vi "Get Channel Name.vi"(8 "error in (no error)":errorcluster, 10 "index":i32, 11 "Impulse Data in":T1) -> (0 "error out":errorcluster, 2 "Channel Name":string, 3 "Impulse Data out":T1)   [LabVIEW 2016, in "Impulse Data.lvclass"]
uses:
  Impulse Data.lvclass
  Instance handle.ctl
  Impulse Data.lvclass/Impulse Data.ctl
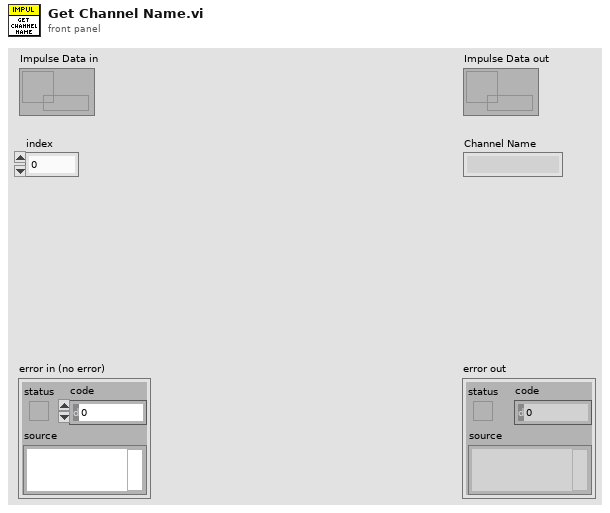
[diagram p1: front panel]
types:
  T1 = typedef "Impulse Data.lvclass/Instance handle.ctl" = refnum<data-value>
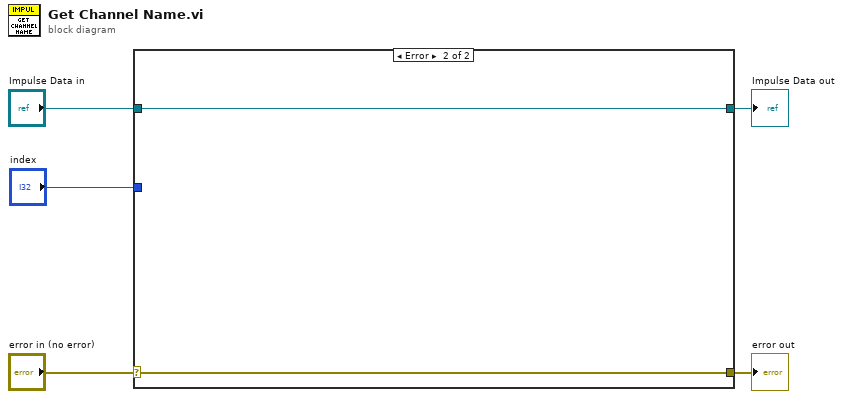
[diagram p0: block diagram]
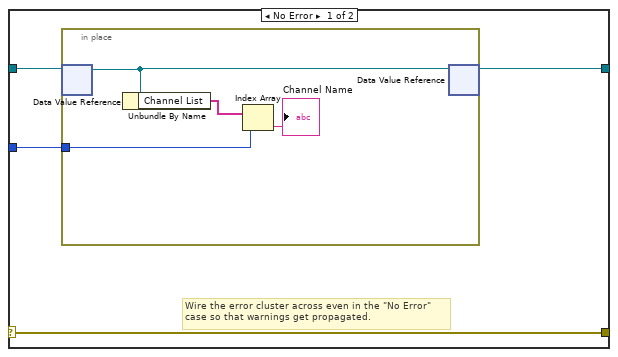
[diagram p2: hidden frame]
diagram:
  n1 = case shown="Error" "error in (no error)" {
    selector: "error in (no error)" -> [w9 w15]
    tunnel: [w9 w15] -> w4
    tunnel: "index" -> [w8 _]
    tunnel: [w7 w14] -> w2
    tunnel: "Impulse Data in" -> [w6 w14]
    frame No Error {
      # "Wire the error cluster across even in the \"No Error\"\ncase so that warnings get propagated."
      n2 = in-place {
        in-place-border: w8 -> [w12]
        n3 = in-place-dvr #1(w6) -> (w10:refnum<class "Impulse Data.lvclass">)  [unwired: 1 out]
        n4 = Unbundle By Name(w10) -> ("Channel List"=w13:string[])
        n5 = Index Array(array=w13, index=w12) -> (element=→"Channel Name":string)
        n6 = in-place-dvr #1(w10) -> (w7:T1)  [unwired: 1 out]
      }
    }
    frame Error {
    }
  }
  "error out" <- w4
  "Impulse Data out" <- w2
